vi "HW_Stream_raw_data_channel.vi"(8 "error in":errorcluster, 10 "Data flow controls in":T2, 11 "VISA resource name in":refnum<visa-resource-name>) -> (0 "error out":errorcluster, 1 "High-speed channel":T1, 2 "Data flow controls out":T2, 3 "VISA resource name out":refnum<visa-resource-name>, 4 "Timestamp":timestamp, 5 "Read buffer (for reference only, data is queued)":string)   [LabVIEW 2018, in "Tracker.lvlib"]
uses:
  Tracker.lvlib
  <extravilib>/ChannelInstances/High Speed Stream-c(str,stamp)/)Channel.ctl
  <vilib>/Instr/_visa.llb/VISA Flush IO Buffer Mask.ctl
  <vilib>/Instr/_visa.llb/Select Event Type.ctl
  <extravilib>/ChannelInstances/High Speed Stream-c(str,stamp).lvlib
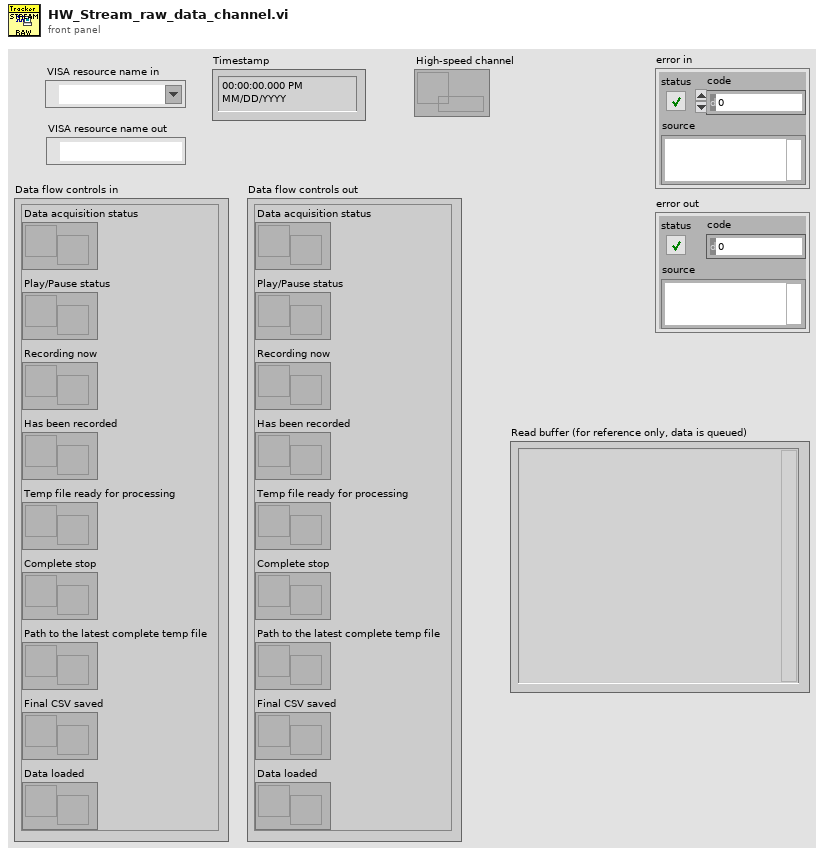
[diagram p1: front panel]
types:
  T1 = typedef "High Speed Stream-c(str,stamp).lvlib/)Channel.ctl" = refnum<queue>
  T2 = cluster{"Data acquisition status":refnum<notifier>, "Play/Pause status":refnum<notifier>, "Complete stop":refnum<notifier>, "Temp file ready for processing":refnum<notifier>, "Has been recorded":refnum<notifier>, "Recording now":refnum<notifier>, "Path to the latest complete temp file":refnum<notifier>, "Final CSV saved":refnum<notifier>, "Data loaded":refnum<notifier>}
  T3 = typedef "VISA Flush IO Buffer Mask.ctl" = u16
  T4 = typedef "Select Event Type.ctl" = u32
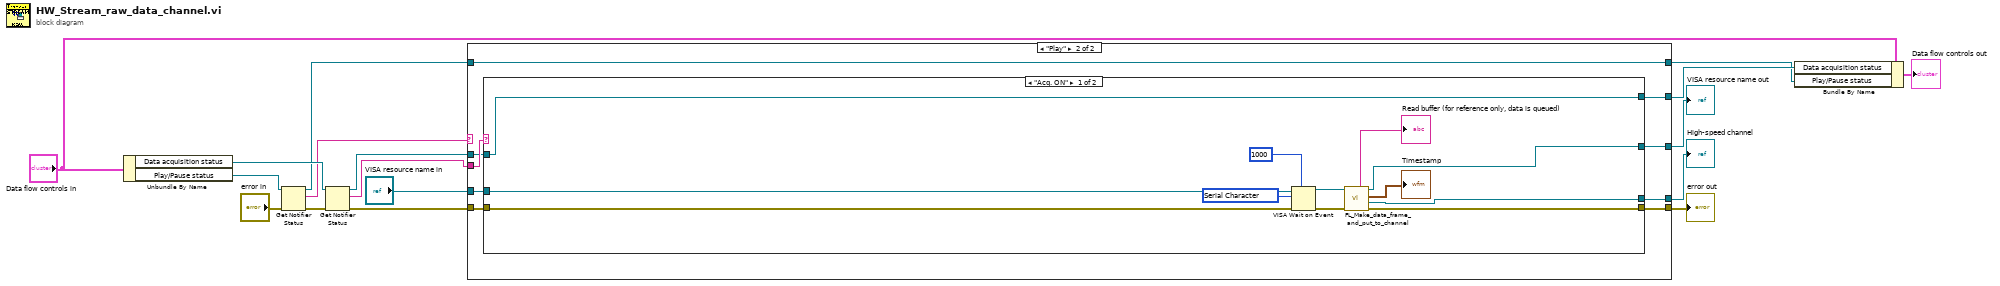
[diagram p0: block diagram]
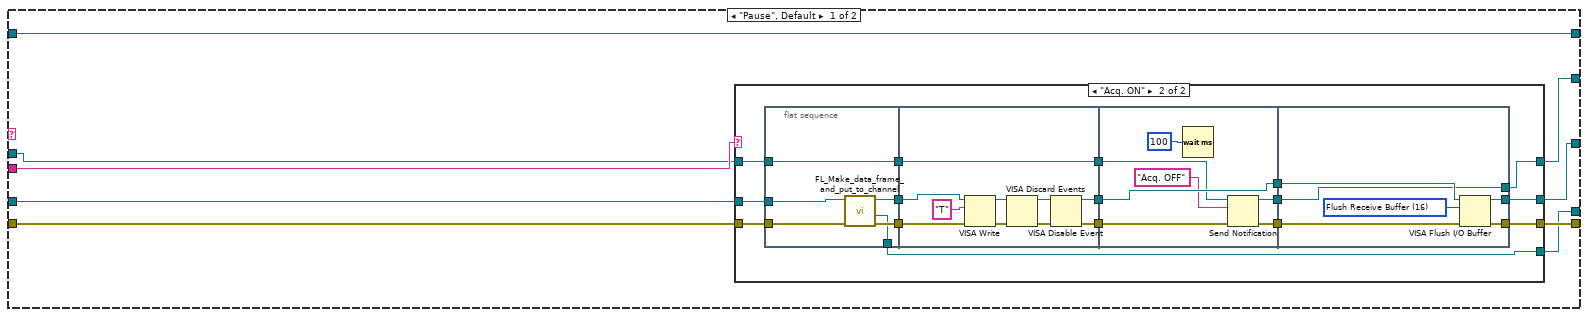
[diagram p2: hidden frame]
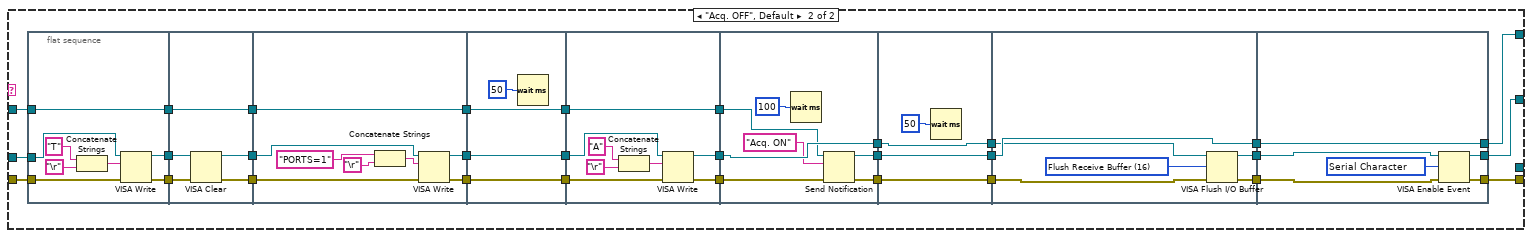
[diagram p4: hidden frame]
diagram:
  n1 = Unbundle By Name("Data flow controls in") -> ("Data acquisition status"=w15:refnum<notifier>, "Play/Pause status"=w14:refnum<notifier>)
  n2 = Get Notifier Status(notifier=w14, error in (no error)="error in") -> (notifier out=w9:refnum<notifier>, current notification=w13:string, error out=w10:errorcluster)  [unwired: 2 out]
  n3 = Get Notifier Status(notifier=w15, error in (no error)=w10) -> (notifier out=w8:refnum<notifier>, current notification=w12:string, error out=w3:errorcluster)  [unwired: 2 out]
  n4 = case shown="\"Play\"" w13 {
    tunnel: [w21 w78] -> w16
    tunnel: "VISA resource name in" -> [w26 w83]
    tunnel: w12 -> [w25 w81]
    tunnel: w9 -> [w23 w79]
    tunnel: w8 -> [w24 w80]
    tunnel: [w20 w77] -> w6
    tunnel: [w23 w79] -> w5
    tunnel: w3 -> [w22 w82]
    tunnel: [w19 w76] -> w2
    tunnel: [w18 w75] -> w1
    frame "Pause", Default {
      n5 = case shown="\"Acq. ON\"" w25 {
        tunnel: w26 -> [w29 w43]
        tunnel: [w29 w42] -> w21
        tunnel: w24 -> [w28 w36]
        tunnel: [w28 w35] -> w20
        tunnel: w22 -> [w27 w39]
        tunnel: [w27 w38] -> w19
        tunnel: [_ w30] -> w18
        frame "Acq. OFF", Default {
        }
        frame "Acq. ON" {
          n6 = flat-sequence {
            tunnel: w36 -> [w51]
            tunnel: w39 -> [w50]
            tunnel: w43 -> [w48]
            tunnel: [w47] -> w33
            tunnel: [w49] -> w32
            tunnel: [w51] -> w31
            tunnel: [w46] -> w30
            tunnel: [w53] -> w45
            tunnel: [w52] -> w44
            tunnel: [w61] -> w37
            tunnel: w33 -> [w59]
            tunnel: w32 -> [w58]
            tunnel: w31 -> [w61]
            tunnel: w45 -> [w67]
            tunnel: w44 -> [w66]
            tunnel: [w67] -> w41
            tunnel: [w65] -> w40
            tunnel: w37 -> [w63]
            tunnel: [w62] -> w34
            tunnel: [w72] -> w42
            tunnel: w41 -> [w73]
            tunnel: w40 -> [w74]
            tunnel: [w70] -> w38
            tunnel: [w69] -> w35
            tunnel: w34 -> [w69]
            frame #0 {
              n7 = call "FL_Make_data_frame_and_put_to_channel.vi"("error in"=w50, "VISA resource name in"=w48) -> ("error out"=w49:errorcluster, "High-speed channel"=w46:T1, "VISA resource name out"=w47:refnum<visa-resource-name>)  [unwired: 5 in, 2 out]
            }
            frame #1 {
              n8 = VISA Write(VISA resource name=w59, write buffer="T", error in (no error)=w58) -> (VISA resource name out=w56:refnum<visa-resource-name>, error out=w57:errorcluster)  [unwired: 1 out]
              n9 = VISA Discard Events(8:w57, 11:w56) -> (0:w55:errorcluster, 3:w54:refnum<visa-resource-name>)  [unwired: 2 in]
              n10 = VISA Disable Event(8:w55, 11:w54) -> (0:w52:errorcluster, 3:w53:refnum<visa-resource-name>)  [unwired: 2 in]
            }
            frame #2 {
              n11 = Wait (ms)(milliseconds to wait=u32 100) -> ()  [unwired: 1 out]
              n12 = Send Notification(notification="Acq. OFF", notifier=w63, error in (no error)=w66) -> (notifier out=w62:refnum<notifier>, error out=w65:errorcluster)
            }
            frame #3 {
              w71 = T3 16 items=["Flush Receive Buffer"=16, "Write Transmit Buffer to Device"=32, "Flush Receive Buffer (No I/O)"=64, "Flush Transmit Buffer"=128] ("Mask")
              n13 = VISA Flush I/O Buffer(VISA resource name=w73, mask (16)=w71, error in (no error)=w74) -> (VISA resource name out=w72:refnum<visa-resource-name>, error out=w70:errorcluster)
            }
          }
        }
      }
    }
    frame "Play" {
      n14 = case shown="\"Acq. ON\"" w81 {
        tunnel: w83 -> [w87 w123]
        tunnel: [w91 w96] -> w78
        tunnel: [w92 w97] -> w76
        tunnel: w82 -> [w89 w116]
        tunnel: w80 -> [w95 w111]
        tunnel: [w95 w110] -> w77
        tunnel: [w90 _] -> w75
        frame "Acq. ON" {
          w84 = T4 1073684533 items=["Service Request"=1073684491, "Trigger"=3221168138, "Clear"=1073684493, "VXI Signal"=1073684512, "VXI/VME Interrupt"=3221168161, "VXI/VME Sysfail"=1073684509, "VXI/VME Sysreset"=1073684510, "GPIB CIC"=1073684498, "GPIB Talk"=1073684499, "GPIB Listen"=1073684500, "PXI Interrupt"=1073684514, "Serial Break"=1073684515, "Serial TermChar"=1073684516, "Serial CTS"=1073684521, "Serial DSR"=1073684522, "Serial DCD"=1073684524, "Serial RI"=1073684526, "Serial Character"=1073684533, "USB Interrupt"=1073684535, "All Enabled"=1073709055] ("Event Type")
          n15 = VISA Wait on Event(7:u32 1000 ("timeout (0)"), 8:w89, 10:w84, 11:w87) -> (0:w88:errorcluster, 3:w86:refnum<visa-resource-name>)  [unwired: 1 in, 2 out]
          n16 = call "FL_Make_data_frame_and_put_to_channel.vi"("error in"=w88, "VISA resource name in"=w86) -> ("error out"=w92:errorcluster, "High-speed channel"=w90:T1, "Timestamp"=→"Timestamp":timestamp, "VISA resource name out"=w91:refnum<visa-resource-name>, "Read buffer (for reference only, data is queued)"=→"Read buffer (for reference only, data is queued)":string)  [unwired: 5 in]
        }
        frame "Acq. OFF", Default {
          n17 = flat-sequence {
            tunnel: w123 -> [w132]
            tunnel: [w133] -> w122
            tunnel: [w131] -> w121
            tunnel: w116 -> [w127]
            tunnel: [w126] -> w112
            tunnel: w111 -> [w126]
            tunnel: [w138] -> w118
            tunnel: [w137] -> w117
            tunnel: w121 -> [w136]
            tunnel: w122 -> [w135]
            tunnel: [w134] -> w113
            tunnel: w112 -> [w134]
            tunnel: w118 -> [w144]
            tunnel: [w143] -> w120
            tunnel: w117 -> [w142]
            tunnel: [w141] -> w119
            tunnel: [w139] -> w114
            tunnel: w113 -> [w139]
            tunnel: [w149] -> w103
            tunnel: [w148] -> w102
            tunnel: [w150] -> w101
            tunnel: w114 -> [w150]
            tunnel: w120 -> [w149]
            tunnel: w119 -> [w148]
            tunnel: [w153] -> w125
            tunnel: [w152] -> w124
            tunnel: w103 -> [w155]
            tunnel: w102 -> [w154]
            tunnel: [w151] -> w115
            tunnel: w101 -> [w151]
            tunnel: w125 -> [w163]
            tunnel: w124 -> [w164]
            tunnel: w115 -> [w161]
            tunnel: [w162] -> w109
            tunnel: [w164] -> w108
            tunnel: [w160] -> w107
            tunnel: w109 -> [w169]
            tunnel: [w169] -> w106
            tunnel: w108 -> [w168]
            tunnel: [w168] -> w105
            tunnel: w107 -> [w167]
            tunnel: [w167] -> w104
            tunnel: w104 -> [w171]
            tunnel: w105 -> [w170]
            tunnel: w106 -> [w172]
            tunnel: [w174] -> w100
            tunnel: [w175] -> w99
            tunnel: [w171] -> w98
            tunnel: [w181] -> w110
            tunnel: w100 -> [w179]
            tunnel: w99 -> [w178]
            tunnel: w98 -> [w181]
            tunnel: [w180] -> w97
            tunnel: [w177] -> w96
            frame #0 {
              n18 = Concatenate Strings("T" ("write buffer"), "\r") -> (w128:string)
              n19 = VISA Write(VISA resource name=w132, write buffer=w128, error in (no error)=w127) -> (VISA resource name out=w133:refnum<visa-resource-name>, error out=w131:errorcluster)  [unwired: 1 out]
            }
            frame #1 {
              n20 = VISA Clear(VISA resource name=w135, error in (no error)=w136) -> (VISA resource name out=w138:refnum<visa-resource-name>, error out=w137:errorcluster)
            }
            frame #2 {
              n21 = Concatenate Strings("PORTS=1" ("write buffer"), "\r") -> (w145:string)
              n22 = VISA Write(VISA resource name=w144, write buffer=w145, error in (no error)=w142) -> (VISA resource name out=w143:refnum<visa-resource-name>, error out=w141:errorcluster)  [unwired: 1 out]
            }
            frame #3 {
              n23 = Wait (ms)(milliseconds to wait=u32 50) -> ()  [unwired: 1 out]
            }
            frame #4 {
              n24 = Concatenate Strings("A" ("write buffer"), "\r") -> (w156:string)
              n25 = VISA Write(VISA resource name=w155, write buffer=w156, error in (no error)=w154) -> (VISA resource name out=w152:refnum<visa-resource-name>, error out=w153:errorcluster)  [unwired: 1 out]
            }
            frame #5 {
              n26 = Wait (ms)(milliseconds to wait=u32 100) -> ()  [unwired: 1 out]
              n27 = Send Notification(notification="Acq. ON", notifier=w161, error in (no error)=w163) -> (notifier out=w160:refnum<notifier>, error out=w162:errorcluster)
            }
            frame #6 {
              n28 = Wait (ms)(milliseconds to wait=u32 50) -> ()  [unwired: 1 out]
            }
            frame #7 {
              w173 = T3 16 items=["Flush Receive Buffer"=16, "Write Transmit Buffer to Device"=32, "Flush Receive Buffer (No I/O)"=64, "Flush Transmit Buffer"=128] ("Mask")
              n29 = VISA Flush I/O Buffer(VISA resource name=w170, mask (16)=w173, error in (no error)=w172) -> (VISA resource name out=w175:refnum<visa-resource-name>, error out=w174:errorcluster)
            }
            frame #8 {
              w176 = T4 1073684533 items=["Service Request"=1073684491, "Trigger"=3221168138, "Clear"=1073684493, "VXI Signal"=1073684512, "VXI/VME Interrupt"=3221168161, "VXI/VME Sysfail"=1073684509, "VXI/VME Sysreset"=1073684510, "GPIB CIC"=1073684498, "GPIB Talk"=1073684499, "GPIB Listen"=1073684500, "PXI Interrupt"=1073684514, "Serial Break"=1073684515, "Serial TermChar"=1073684516, "Serial CTS"=1073684521, "Serial DSR"=1073684522, "Serial DCD"=1073684524, "Serial RI"=1073684526, "Serial Character"=1073684533, "USB Interrupt"=1073684535, "All Enabled"=1073709055] ("Event Type")
              n30 = VISA Enable Event(8:w179, 10:w176, 11:w178) -> (0:w180:errorcluster, 3:w177:refnum<visa-resource-name>)  [unwired: 1 in]
            }
          }
        }
      }
    }
  }
  "VISA resource name out" <- w16
  "error out" <- w2
  "High-speed channel" <- w1
  n31 = Bundle By Name(cluster="Data flow controls in", "Data acquisition status"=w6, "Play/Pause status"=w5) -> (→"Data flow controls out":T2)
